vi "Obtain Queue.vi"(8 "error in (no error)":errorcluster, 10 "Queue Name":string, 11 "VI Refnum":refnum<vi>) -> (0 "error out":errorcluster, 3 "Message Queue":T1)   [LabVIEW 2019, in "Acquire Mouse.lvlib"]
doc: "Function to enqueue a Message in a Queue of other Module."
uses:
  Acquire Mouse.lvlib
  Shared/TypeDefs/Message Queue Ref.ctl
  Shared/TypeDefs/Message Queue Type.ctl
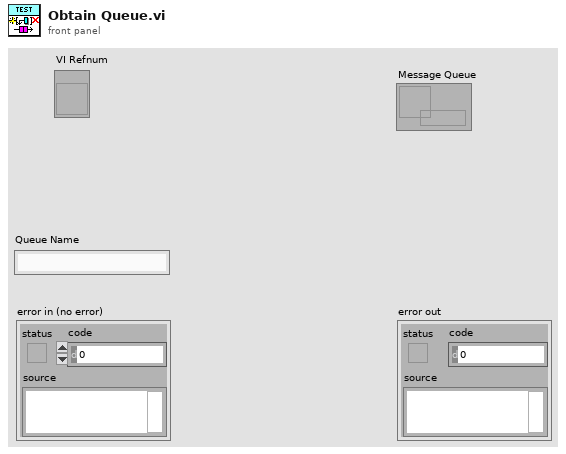
[diagram p1: front panel]
types:
  T1 = typedef "Message Queue Ref.ctl" = refnum<queue>
  T2 = typedef "Message Queue Type.ctl" = cluster{"Custom State Name":string, "Defined State Name":variant, "Call Chain":string[], "Message Data":variant}
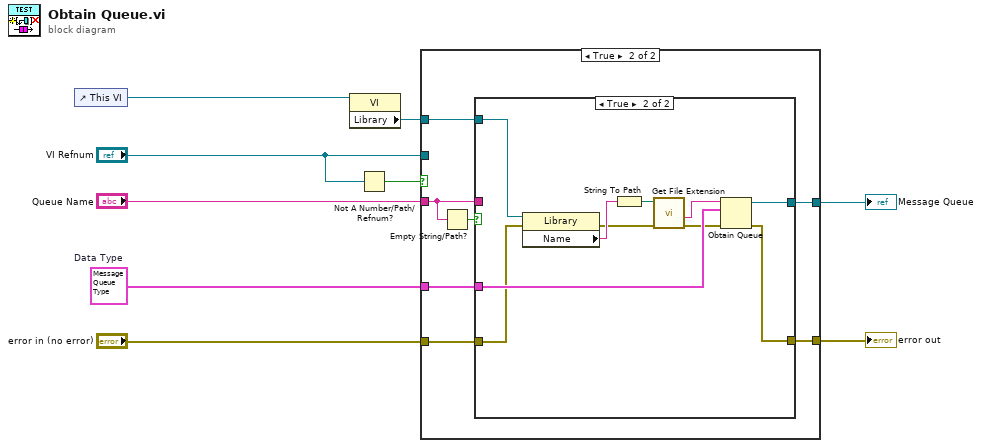
[diagram p0: block diagram]
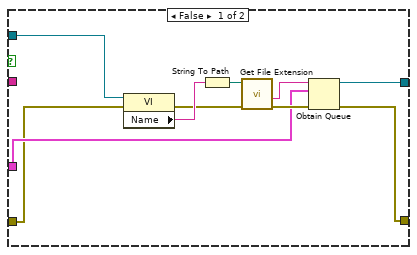
[diagram p2: hidden frame]
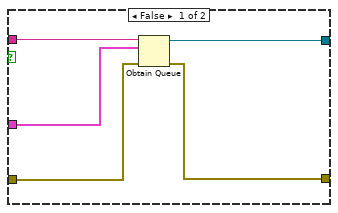
[diagram p3: hidden frame]
diagram:
  w1 = T2 {"Custom State Name"="", "Defined State Name"=variant(enum16{"Initialize", "Re-Initialize", "Initialize Data", "Initialize Panel", "[Event Structure] Update Data", "Add VI", "Get Splitters", "Map Splitter Pos to Coords", "Initialize Mouse", "Acquire Data", "Process Data", "Error", "Exit", "Default"} enum."Initialize"), "Call Chain"=[], "Message Data"=variant}  # Data Type
  n1 = control-ref of="This VI"() -> (w6:refnum<vi>)
  n2 = property class="VI"(reference=w6) -> ("Library"=w5:refnum<vi>)  [unwired: 1 in, 2 out]
  n3 = Not A Number/Path/Refnum?(number/path/refnum="VI Refnum") -> (NaN/Path/Refnum?=w3:bool)
  n4 = case shown="True" w3 {
    tunnel: "Queue Name" -> [_ w25]
    tunnel: w1 -> [w13 w24]
    tunnel: [w11 w23] -> w8
    tunnel: "error in (no error)" -> [w10 w22]
    tunnel: [w12 w21] -> w2
    tunnel: w5 -> [_ w20]
    tunnel: "VI Refnum" -> [w14 _]
    frame False {
      n5 = property class="VI"(reference=w14, error in=w10) -> (error out=w16:errorcluster, "Name"=w18:string)  [unwired: 1 out]
      n6 = String To Path(string=w18) -> (path=w17:path)
      n7 = call <vilib>:"Get File Extension.vi"("error in (no error)"=w16, "file"=w17) -> ("error out"=w15:errorcluster, "filename without extension"=w19:string)  [unwired: 8 out]
      n8 = Obtain Queue(name (unnamed)=w19, element data type=w13, error in (no error)=w15) -> (queue out=w12:refnum<queue>, error out=w11:errorcluster)  [unwired: 2 in, 1 out]
    }
    frame True {
      n9 = Empty String/Path?(string/path=w25) -> (empty?=w26:bool)
      n10 = case shown="True" w26 {
        tunnel: w22 -> [w31 w34]
        tunnel: [w30 w41] -> w23
        tunnel: [w29 w40] -> w21
        tunnel: w25 -> [w28 _]
        tunnel: w24 -> [w27 w39]
        tunnel: w20 -> [_ w38]
        frame False {
          n11 = Obtain Queue(name (unnamed)=w28, element data type=w27, error in (no error)=w31) -> (queue out=w29:refnum<queue>, error out=w30:errorcluster)  [unwired: 2 in, 1 out]
        }
        frame True {
          n12 = property class="Library"(reference=w38, error in=w34) -> (error out=w33:errorcluster, "Name"=w36:string)  [unwired: 1 out]
          n13 = String To Path(string=w36) -> (path=w35:path)
          n14 = call <vilib>:"Get File Extension.vi"("error in (no error)"=w33, "file"=w35) -> ("error out"=w32:errorcluster, "filename without extension"=w37:string)  [unwired: 8 out]
          n15 = Obtain Queue(name (unnamed)=w37, element data type=w39, error in (no error)=w32) -> (queue out=w40:refnum<queue>, error out=w41:errorcluster)  [unwired: 2 in, 1 out]
        }
      }
    }
  }
  "error out" <- w8
  "Message Queue" <- w2
